vi "Update RPC Client Method Constants.vi"(5 "Server class in":refnum<vi>, 7 "RPC Method Parameters":T1[](array[typedef]), 8 "error in (no error)":errorcluster, 10 "RPC Method Name":string, 11 "VI in":refnum<vi>) -> (0 "error out":errorcluster, 3 "VI out":refnum<vi>)   [LabVIEW 2019, in "gRPC Scripting Tools.lvlib"]
uses:
  gRPC Scripting Tools.lvlib
  TypeDefs/RPC Method Parameters.ctl
  <vilib>/Utility/traverseref.llb/TRef TravTarget.ctl
  0eaa7444-8baf-4465-b530-593cae42fb70.vi
  <vilib>/Comparison/Equal/Equal Functor/Equal Functor.lvclass
  <vilib>/Utility/traverseref.llb/VI Scripting - Traverse.lvlib
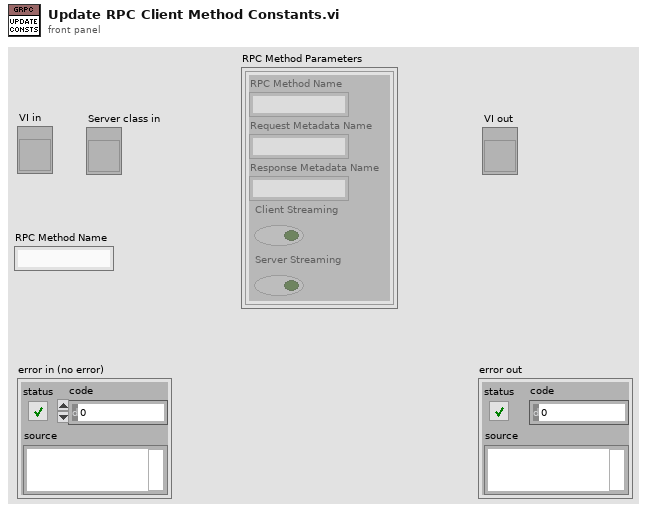
[diagram p1: front panel]
types:
  T1 = typedef "gRPC Scripting Tools.lvlib/RPC Method Parameters.ctl" = cluster{"RPC Method Name":string, "Request Metadata Name":string, "Response Metadata Name":string, "Client Streaming":bool, "Server Streaming":bool}
  T2 = typedef "TRef TravTarget.ctl" = enum16{"FP", "BD", "Other"}
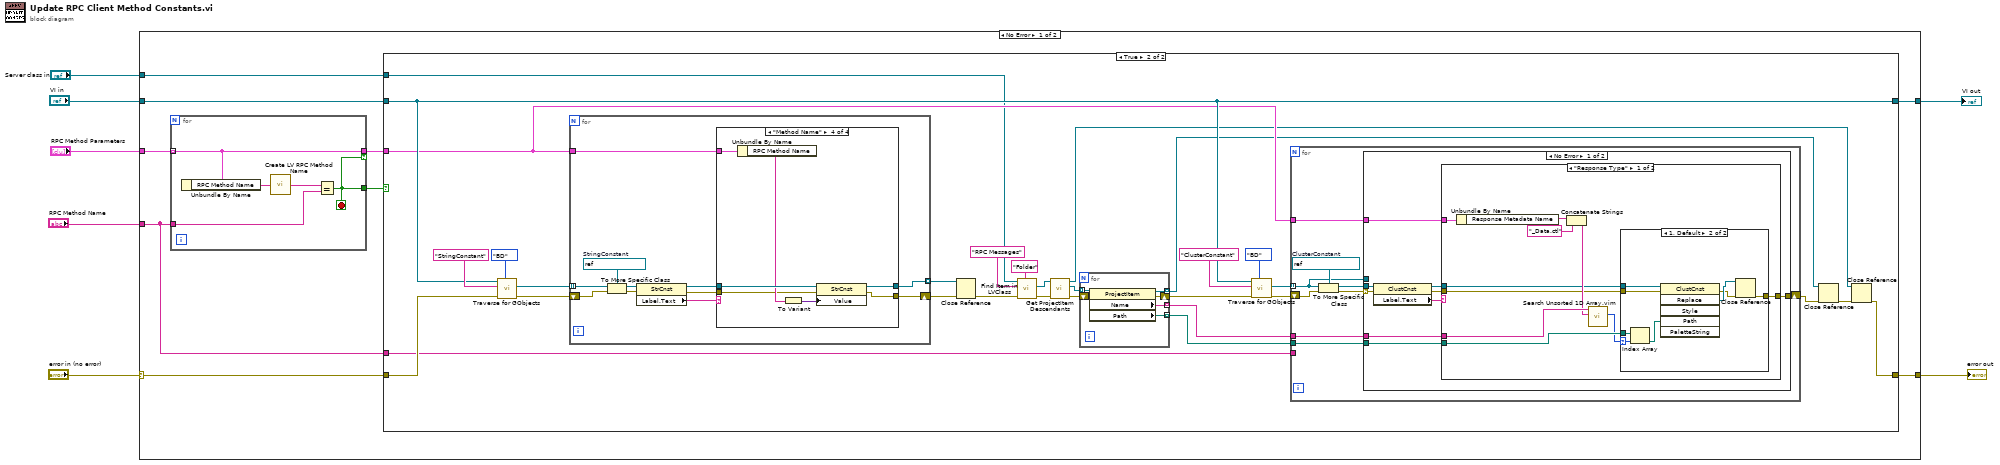
[diagram p0: block diagram]
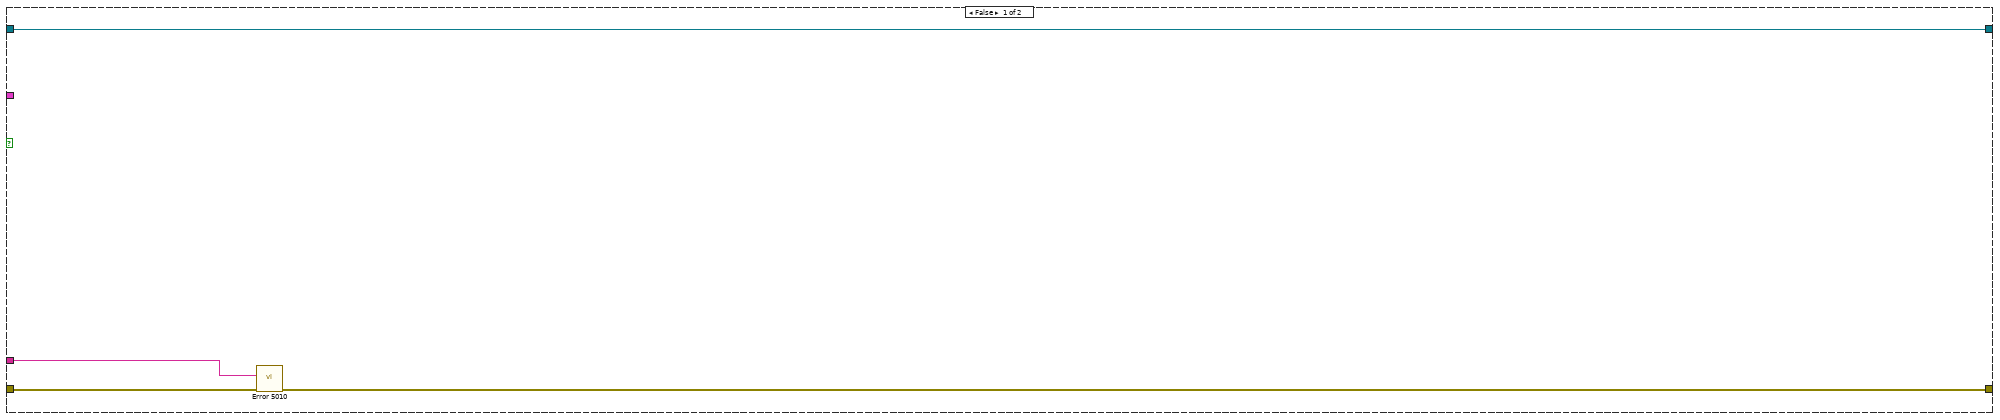
[diagram p2: hidden frame]
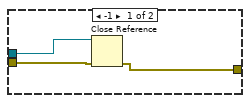
[diagram p3: hidden frame]
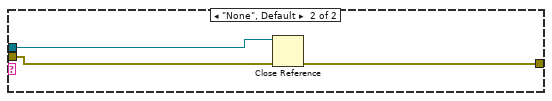
[diagram p4: hidden frame]
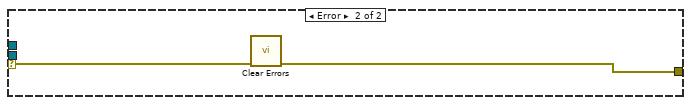
[diagram p5: hidden frame]
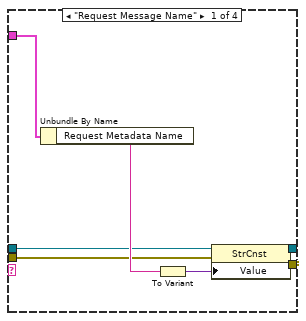
[diagram p6: hidden frame]
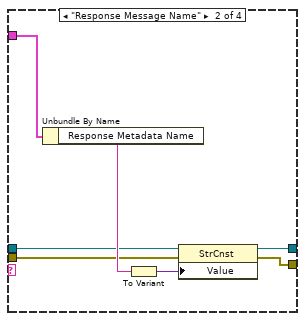
[diagram p7: hidden frame]
diagram:
  n1 = case shown="No Error" "error in (no error)" {
    selector: "error in (no error)" -> [w11 w141]
    tunnel: [w16 w141] -> w7
    tunnel: "VI in" -> [w15 w140]
    tunnel: "RPC Method Parameters" -> [w14 _]
    tunnel: "RPC Method Name" -> [w9 _]
    tunnel: [w10 w140] -> w2
    tunnel: "Server class in" -> [w8 _]
    frame No Error {
      n2 = for {
        tunnel: w14 -> [w138] mode=indexing
        tunnel: w9 -> [w139]
        tunnel: [w138] -> w12 if=w137
        tunnel: [w137] -> w13
        stop <- w137 stop-if-true
        n3 = Unbundle By Name(w138) -> ("RPC Method Name"=w136:string)
        n4 = call "Create LV RPC Method Name.vi"("Proto Parser RPC Method Name in"=w136) -> ("LV RPC Method Name out"=w135:string)
        n5 = Equal?(x=w135, y=w139) -> (x = y?=w137:bool)
      }
      n6 = case shown="True" w13 {
        tunnel: [w17 w21] -> w16
        tunnel: w11 -> [w19 w50]
        tunnel: w15 -> [w20 w41]
        tunnel: w12 -> [_ w37]
        tunnel: [w20 w41] -> w10
        tunnel: w9 -> [w18 w38]
        tunnel: w8 -> [_ w28]
        frame False {
          n7 = call "Error 5010.vi"("error in (no error)"=w19, "RPC Method Name"=w18) -> ("error out"=w17:errorcluster)  [unwired: 9 in]
        }
        frame True {
          n8 = call <vilib>:"Traverse for GObjects.vi"("Traverse Target"=TRef_TravTarget."BD", "error in (no error)"=w50, "Class Name"="StringConstant", "VI Refnum"=w41) -> ("error out"=w47:errorcluster, "References"=w43:refnum<vi>[])  [unwired: 4 in, 2 out]
          n9 = for {
            tunnel: w43 -> [w110] mode=indexing
            shift-right: [w102] -> w44
            shift-left: w47 -> [w109]
            tunnel: w37 -> [w105]
            tunnel: [w101] -> w42 mode=indexing
            w111 = refnum<vi> refnum  # StringConstant
            n10 = To More Specific Class(target class=w111, reference=w110, error in=w109) -> (specific class reference=w108:refnum<vi>, error out=w107:errorcluster)
            n11 = property class="StrCnst"(reference=w108, error in=w107) -> (reference out=w104:refnum<vi>, error out=w103:errorcluster, "Label.Text"=w106:string)
            n12 = case shown="\"Method Name\"" w106 {
              tunnel: w105 -> [w113 w123 _ w134]
              tunnel: w104 -> [w115 w121 w126 w133]
              tunnel: w103 -> [w116 w122 w127 w130]
              tunnel: [w114 w120 w127 w129] -> w102
              tunnel: [w112 w119 w126 w128] -> w101
              frame "Request Message Name" {
                n13 = Unbundle By Name(w113) -> ("Request Metadata Name"=w118:string)
                n14 = To Variant(anything=w118) -> (Variant=w117:variant)
                n15 = property class="StrCnst"(reference=w115, error in=w116, "Value"=w117) -> (reference out=w112:refnum<vi>, error out=w114:errorcluster)
              }
              frame "Response Message Name" {
                n16 = Unbundle By Name(w123) -> ("Response Metadata Name"=w125:string)
                n17 = To Variant(anything=w125) -> (Variant=w124:variant)
                n18 = property class="StrCnst"(reference=w121, error in=w122, "Value"=w124) -> (reference out=w119:refnum<vi>, error out=w120:errorcluster)
              }
              frame "None", Default {
              }
              frame "Method Name" {
                n19 = Unbundle By Name(w134) -> ("RPC Method Name"=w132:string)
                n20 = To Variant(anything=w132) -> (Variant=w131:variant)
                n21 = property class="StrCnst"(reference=w133, error in=w130, "Value"=w131) -> (reference out=w128:refnum<vi>, error out=w129:errorcluster)
              }
            }
          }
          n22 = Close Reference(reference=w42, error in (no error)=w44) -> (error out=w31:errorcluster)
          n23 = call "Find Item in LVClass.vi"("Item Type"="Folder", "error in (no error)"=w31, "Item Name"="RPC Messages", "Class Item in"=w28) -> ("error out"=w35:errorcluster, "Project Item (Class Item)"=w34:refnum<vi>)  [unwired: 4 in, 2 out]
          n24 = call "Get ProjectItem Descendants.vi"("error in (no error)"=w35, "ProjectItem in"=w34) -> ("error out"=w30:errorcluster, "All Descendents"=w36:refnum<vi>[], "ProjectItem out"=w27:refnum<vi>)  [unwired: 7 in]
          n25 = for {
            tunnel: w36 -> [w56] mode=indexing
            tunnel: [w55] -> w25 mode=indexing
            tunnel: [w54] -> w24 mode=indexing
            shift-right: [w52] -> w29
            shift-left: w30 -> [w53]
            tunnel: [w51] -> w23 mode=indexing
            n26 = property class="ProjectItem"(reference=w56, error in=w53) -> (reference out=w54:refnum<vi>, error out=w52:errorcluster, "Name"=w55:string, "Path"=w51:path)
          }
          n27 = call <vilib>:"Traverse for GObjects.vi"("Traverse Target"=TRef_TravTarget."BD", "error in (no error)"=w29, "Class Name"="ClusterConstant", "VI Refnum"=w41) -> ("error out"=w40:errorcluster, "References"=w39:refnum<vi>[])  [unwired: 4 in, 2 out]
          n28 = for {
            tunnel: w39 -> [w57] mode=indexing
            shift-right: [w61] -> w26
            shift-left: w40 -> [w64]
            tunnel: w38 -> [_]
            tunnel: w37 -> [w60]
            tunnel: w25 -> [w59]
            tunnel: w23 -> [w58]
            w65 = refnum<vi> refnum  # ClusterConstant
            n29 = To More Specific Class(target class=w65, reference=w57, error in=w64) -> (specific class reference=w63:refnum<vi>, error out=w62:errorcluster)
            n30 = case shown="No Error" w62 {
              selector: w62 -> [w73 w100]
              tunnel: w63 -> [w74 _]
              tunnel: [w69 w99] -> w61
              tunnel: w60 -> [w68 _]
              tunnel: w59 -> [w67 _]
              tunnel: w58 -> [w66 _]
              tunnel: w57 -> [_ _]
              frame No Error {
                n31 = property class="ClustCnst"(reference=w74, error in=w73) -> (reference out=w71:refnum<vi>, error out=w70:errorcluster, "Label.Text"=w72:string)
                n32 = case shown="\"Response Type\"" w72 {
                  tunnel: w71 -> [w77 w98]
                  tunnel: w70 -> [w76 w97]
                  tunnel: [w75 w96] -> w69
                  tunnel: w68 -> [w84 _]
                  tunnel: w67 -> [w81 _]
                  tunnel: w66 -> [w79 _]
                  frame "Response Type" {
                    n33 = Unbundle By Name(w84) -> ("Response Metadata Name"=w83:string)
                    n34 = Concatenate Strings(w83, "_Data.ctl" ("string")) -> (w80:string)
                    n35 = call "Search Unsorted 1D Array.vim"("element"=w80, "unsorted 1D array"=w81) -> ("index of element"=w78:i32)  [unwired: 9 in]
                    n36 = case shown="1, Default" w78 {
                      selector: w78 -> [_ w94]
                      tunnel: w79 -> [_ w95]
                      tunnel: w77 -> [w87 w93]
                      tunnel: w76 -> [w86 w92]
                      tunnel: [w85 w88] -> w75
                      frame -1 {
                        n37 = Close Reference(reference=w87, error in (no error)=w86) -> (error out=w85:errorcluster)
                      }
                      frame 1, Default {
                        n38 = Index Array(array=w95, index=w94) -> (element=w91:path)
                        n39 = invoke class="ClustCnst" method="Replace"(reference=w93, error in=w92, "Path"=w91) -> (error out=w89:errorcluster, "Replace"=w90:refnum<vi>)  [unwired: 3 in, 4 out]
                        n40 = Close Reference(reference=w90, error in (no error)=w89) -> (error out=w88:errorcluster)
                      }
                    }
                  }
                  frame "None", Default {
                    n41 = Close Reference(reference=w98, error in (no error)=w97) -> (error out=w96:errorcluster)
                  }
                }
              }
              frame Error {
                n42 = call <vilib>:"Clear Errors.vi"("error in (no error)"=w100) -> ("error out"=w99:errorcluster)  [unwired: 5 in, 1 out]
              }
            }
          }
          n43 = Close Reference(reference=w24, error in (no error)=w26) -> (error out=w22:errorcluster)
          n44 = Close Reference(reference=w27, error in (no error)=w22) -> (error out=w21:errorcluster)
        }
      }
    }
    frame Error {
    }
  }
  "error out" <- w7
  "VI out" <- w2
